vi "CC_IO_tcp.vi"(3 "error in (no error) 2":errorcluster, 4 "Command":string, 5 "connection ID":refnum<k5>) -> (0 "error out 2":errorcluster, 1 "Response":string, 2 "connection ID out":refnum<k5>)   [LabVIEW 2019]
doc: "Cryocon Output then Input VI.\nWrites a command string to an open instrument, then reads the response.\nThe ERROR VI is called to handle any input/output errors."
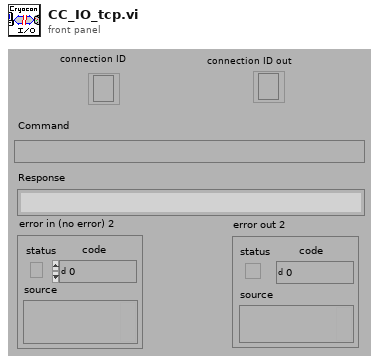
[diagram p1: front panel]
types:
  T1 = enum16{"Standard", "Buffered", "CRLF", "Immediate"}
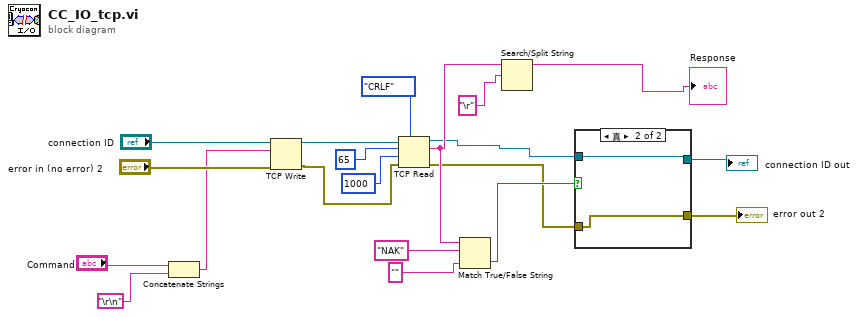
[diagram p0: block diagram]
diagram:
  n1 = Concatenate Strings("Command", "\r\n") -> (w6:string)
  n2 = TCP Write(connection ID="connection ID", data in=w6, error in (no error)="error in (no error) 2") -> (connection ID out=w10:refnum<k5>, error out=w16:errorcluster)  [unwired: 1 in, 1 out]
  n3 = TCP Read(connection ID=w10, bytes to read=65, error in (no error)=w16, 7:T1."CRLF" ("mode (standard)"), 9:1000 ("timeout ms (25000)")) -> (connection ID out=w2:refnum<k5>, data out=w5:string, error out=w1:errorcluster)
  n4 = Match True/False String(2:"", 3:"NAK", 4:w5) -> (0:w12:bool)  [unwired: 1 out]
  n5 = Search/Split String(string=w5, search string/char (-)="\r") -> (substring before match=→"Response":string)  [unwired: 1 in, 2 out]
  n6 = case shown="真" w12 {
    tunnel: w1 -> [w21 w23]
    tunnel: w2 -> [w22 w24]
    tunnel: [w22 w24] -> w14
    tunnel: [w21 w23] -> w13
    frame False {
    }
    frame True {
    }
  }
  "error out 2" <- w13
  "connection ID out" <- w14
